vi "Close.vi"(8 "error in (no error)":errorcluster, 11 "SigGen_NIRF in":refnum<class "SigGen_NIRF.lvclass">) -> (0 "error out":errorcluster)   [LabVIEW 2014, in "SigGen_NIRF.lvclass"]
uses:
  SigGen_NIRF.lvclass
  SigGen_NIRF.lvclass/SigGen_NIRF.ctl
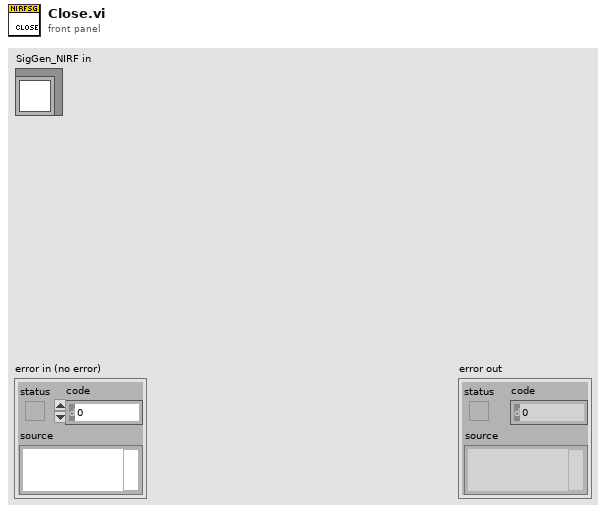
[diagram p1: front panel]
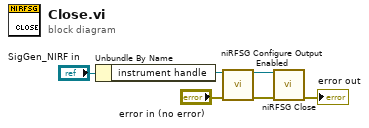
[diagram p0: block diagram]
diagram:
  n1 = Unbundle By Name("SigGen_NIRF in") -> ("instrument handle"=w4:refnum<k15>)
  n2 = call <instrlib>:"niRFSG Configure Output Enabled.vi"("instrument handle"=w4, "error in"="error in (no error)") -> ("instrument handle out"=w3:refnum<k15>, "error out"=w2:errorcluster)  [unwired: 12 in]
  n3 = call <instrlib>:"niRFSG Close.vi"("instrument handle"=w3, "error in"=w2) -> ("error out"=→"error out":errorcluster)  [unwired: 13 in]
